vi "Get T_0 Index.vi"(8 "error in (no error)":errorcluster, 11 "task/channels in":refnum<k21>="PrecorAI") -> (0 "error out":errorcluster, 1 "Num TCs":i32, 2 "Index of Temperature Channel 0":i32, 3 "task/channels out":refnum<k21>, 4 "All channels":string[](array[string]), 5 "Non-TC Channels":refnum<k21>[](array[refnum]))   [LabVIEW 2017]
uses:
  <resource>/objmgr/daqmx.rc
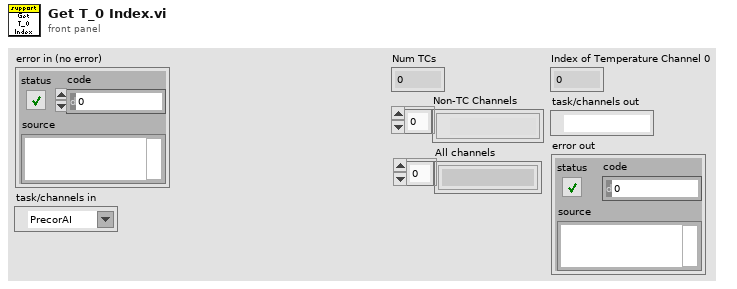
[diagram p1: front panel]
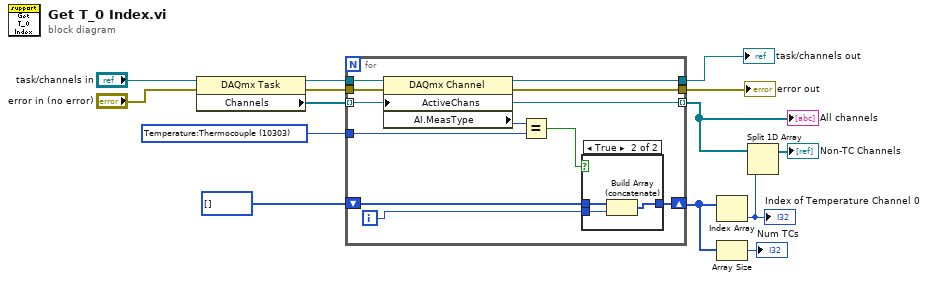
[diagram p0: block diagram]
diagram:
  w9 = 10303 items=["Voltage"=10322, "Voltage RMS"=10350, "Current"=10134, "Current RMS"=10351, "More:Voltage:Custom with Excitation"=10323, "More:Bridge (V/V)"=15908, "Frequency"=10181, "Resistance"=10278, "Temperature:Thermocouple"=10303, "Temperature:Thermistor"=10302, "Temperature:RTD"=10301, "Temperature:Built-in Sensor"=10311, "Strain Gage"=10300, "Rosette Strain Gage"=15980, "Position:LVDT"=10352, "Position:RVDT"=10353, "Position:Eddy Current Proximity Probe"=14835, "Accelerometer"=10356, "Velocity:IEPE Sensor"=15966, "Force:Bridge"=15899, "Force:IEPE Sensor"=15895, "Pressure:Bridge"=15902, "Sound Pressure:Microphone"=10354, "Torque:Bridge"=15905, "TEDS Sensor"=12531] ("AI.MeasType")
  n1 = property class="DAQmx Task"(reference="task/channels in", error in="error in (no error)") -> (reference out=w12:refnum<k21>, error out=w11:errorcluster, "Channels"=w13:refnum<k21>[])
  n2 = for {
    tunnel: w13 -> [w15] mode=indexing
    tunnel: w12 -> [w25]
    tunnel: w11 -> [w24]
    tunnel: w9 -> [w23]
    tunnel: [w22] -> w8
    tunnel: [w21] -> w7
    shift-right: [w18] -> w5
    shift-left: i32[] [] -> [w19]
    tunnel: [w15] -> w1 mode=indexing
    i -> [w16]
    n3 = property class="DAQmx Channel"(reference=w25, error in=w24, "ActiveChans"=w15) -> (reference out=w22:refnum<k21>, error out=w21:errorcluster, "AI.MeasType"=w17:i32)
    n4 = Equal?(x=w17, y=w23) -> (x = y?=w20:bool)
    n5 = case shown="True" w20 {
      tunnel: w19 -> [w26 w29]
      tunnel: [w26 w28] -> w18
      tunnel: w16 -> [_ w27]
      frame False {
      }
      frame True {
        n6 = Build Array (concatenate)(w29, w27) -> (w28:i32[])
      }
    }
  }
  "task/channels out" <- w8
  "error out" <- w7
  "All channels" <- w1
  n7 = Index Array(array=w5) -> (element=w3:i32)  [unwired: 1 in]
  "Index of Temperature Channel 0" <- w3
  n8 = Array Size(array=w5) -> (size(s)=→"Num TCs":i32)
  n9 = Split 1D Array(array=w1, index=w3) -> (first subarray=→"Non-TC Channels":refnum<k21>[])  [unwired: 1 out]
